vi "Do CW Output.vi"(8 "error in":errorcluster, 9 "Attenuation (0)":dbl, 10 "400 MHz Power (0x1F)":u8=31 format="%02x", 11 "VISA resource":refnum<visa-resource-name>="COM5") -> (0 "error out":errorcluster, 3 "VISA resource dup":refnum<visa-resource-name>)   [LabVIEW 2010]
uses:
  MICS Parameters Global.vi
  MICS_ID Global.vi
panel:
  in  "CAL_400_MHZ_ANT? (FALSE)":bool
  in  "TX Mode (On)":bool=TRUE
  in  "Frequency Range (2.45 GHz)":enum16{"2.45GHz", "400MHz"}(ring)
  in  "2.45 GHz Power (10)":i8(ring)=10 items=["-29"=-29, "-4"=-4, "-2"=-2, "0"=0, "2"=2, "4"=4, "6"=6, "8"=8, "10"=10, "12"=12, "14"=14, "16"=16, "18"=18, "20"=20, "22"=22, "24"=24, "26"=26, "27"=27]
  in  "MICS_Channel (0-9 Inclusive)":u16=2
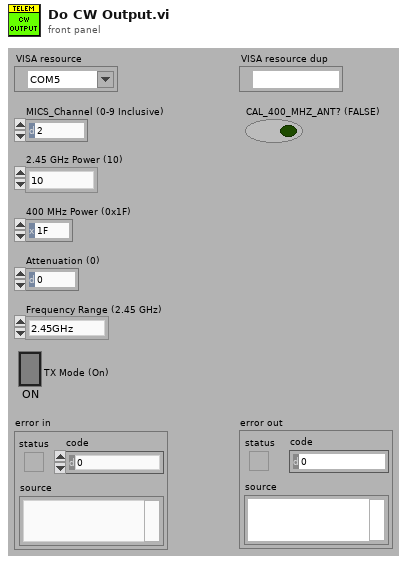
[diagram p1: front panel]
types:
  T1 = cluster{"ConfigFlags":u8, "ImplantID":u32, "CompanyID":u8, "Normal_Comm":cluster{"RF_Channel":u8, "UserData":u8, "TX_Mod":u8, "RX_Mod":u8, "RX_BlockSize":u8, "BlockPerPack":u8, "TX_BlockSize":u8}, "Emerg_Comm":cluster{"RF_Channel":u8, "UserData":u8, "TX_Mod":u8, "RX_Mod":u8, "TX_BlockSize":u8, "BlockPerPack":u8, "RX_BlockSize":u8}, "ImplantRev":u8, "245TX_PowerCal":i8, "245TX_Power":i8, "CCA_RSSI_Thresholds":cluster{"ch0":u16, "ch1":u16, "ch2":u16, "ch3":u16, "ch4":u16, "ch5":u16, "ch6":u16, "ch7":u16, "ch8":u16, "ch9":u16}}
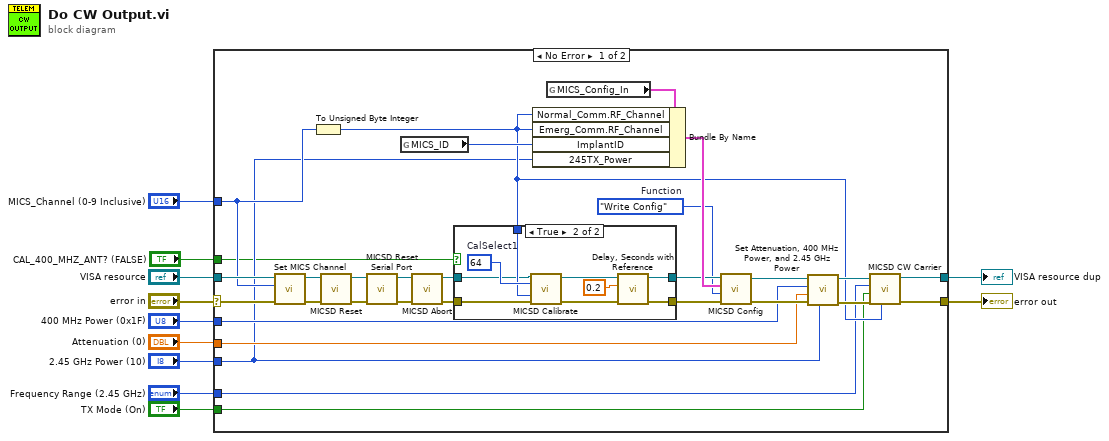
[diagram p0: block diagram]
diagram:
  n1 = case shown="No Error" "error in" {
    selector: "error in" -> [w32 w53]
    tunnel: "400 MHz Power (0x1F)" -> [w27 _]
    tunnel: [w18 w53] -> w10
    tunnel: "VISA resource" -> [w38 w52]
    tunnel: "Attenuation (0)" -> [w28 _]
    tunnel: "MICS_Channel (0-9 Inclusive)" -> [w17 _]
    tunnel: [w20 w52] -> w4
    tunnel: "2.45 GHz Power (10)" -> [w15 _]
    tunnel: "Frequency Range (2.45 GHz)" -> [w14 _]
    tunnel: "TX Mode (On)" -> [w13 _]
    tunnel: "CAL_400_MHZ_ANT? (FALSE)" -> [w12 _]
    frame No Error {
      w26 = enum16{"Write Config", "Read Config"}."Write Config"  # Function
      n2 = call "Set MICS Channel.vi"("error in"=w32, "MICS_Channel"=w17) -> ("error out"=w31:errorcluster)  [unwired: 5 in]
      n3 = To Unsigned Byte Integer(number=w17) -> (unsigned 8bit integer=w16:u8)
      n4 = call "MICSD Reset.vi"("error in (no error)"=w31, "VISA Resource Name"=w38) -> ("error out"=w40:errorcluster, "dup VISA Resource Name"=w39:refnum<visa-resource-name>)  [unwired: 8 in]
      n5 = call "MICSD Reset Serial Port.vi"("error in (no error)"=w40, "VISA Resource Name"=w39) -> ("error out"=w24:errorcluster, "dup VISA Resource Name"=w25:refnum<visa-resource-name>)  [unwired: 8 in]
      n6 = global read "MICS_ID Global.vi" "MICS_ID"() -> (w34:u32)
      n7 = call "MICSD Abort.vi"("error in (no error)"=w24, "VISA Resource Name"=w25) -> ("error out"=w22:errorcluster, "dup VISA Resource Name"=w23:refnum<visa-resource-name>)  [unwired: 8 in]
      n8 = case shown="True" w12 {
        tunnel: [w41 w49] -> w36
        tunnel: [w42 w46] -> w33
        tunnel: w16 -> [_ w45]
        tunnel: w23 -> [w42 w44]
        tunnel: w22 -> [w41 w43]
        frame False {
        }
        frame True {
          w51 = u8 64  # CalSelect1
          n9 = call "MICSD Calibrate.vi"("VISA Resource Name"=w44, "CalSelect1"=w51, "Channel"=w45, "error in (no error)"=w43) -> ("dup VISA Resource Name"=w47:refnum<visa-resource-name>, "error out"=w50:errorcluster)  [unwired: 10 in]
          n10 = call "Delay, Seconds with Reference.vi"("error in"=w50, "delay"=dbl[unit] 0.2, "VISA resource"=w47) -> ("error out"=w49:errorcluster, "VISA resource dup"=w46:refnum<visa-resource-name>)  [unwired: 3 in, 1 out]
        }
      }
      n11 = global read "MICS Parameters Global.vi" "MICS_Config_In"() -> (w35:T1)
      n12 = Bundle By Name(cluster=w35, "Normal_Comm.RF_Channel"=w16, "Emerg_Comm.RF_Channel"=w16, "ImplantID"=w34, "245TX_Power"=w15) -> (w37:T1)
      n13 = call "MICSD Config.vi"("error in (no error)"=w36, "Function"=w26, "MICS_Config_In"=w37, "VISA Resource Name"=w33) -> ("error out"=w29:errorcluster, "dup VISA Resource Name"=w30:refnum<visa-resource-name>)  [unwired: 5 in, 1 out]
      n14 = call "Set Attenuation, 400 MHz Power, and 2.45 GHz Power.vi"("2.45 GHz Power (10)"=w15, "error in"=w29, "Attenuation dB (0)"=w28, "MICS Power Setting (0x1F)"=w27, "VISA Resource Name"=w30) -> ("error out"=w19:errorcluster, "dup VISA Resource Name"=w21:refnum<visa-resource-name>)  [unwired: 5 in]
      n15 = call "MICSD CW Carrier.vi"("400MHz Channel"=w16, "error in (no error)"=w19, "TX Mode (Off)"=w13, "Frequency Range"=w14, "VISA Resource Name"=w21) -> ("error out"=w18:errorcluster, "dup VISA Resource Name"=w20:refnum<visa-resource-name>)  [unwired: 5 in]
    }
    frame Error {
    }
  }
  "error out" <- w10
  "VISA resource dup" <- w4
